vi "PID Get Error (DBL).vi"(0 "setpoint":dbl format="%.2f", 1 "process variable":dbl format="%.2f", 2 "beta":dbl=1.0 format="%.2f", 3 "linearity":dbl=1.0 format="%.2f", 4 "setpoint range":cluster{"setpoint high":dbl, "setpoint low":dbl}={"setpoint high"=100.0, "setpoint low"=0.0} {"setpoint high" format="%.2f"; "setpoint low" format="%.2f"}) -> (5 "error (with beta)":dbl format="%.2f", 6 "error":dbl format="%.2f")   [LabVIEW 2017, in "NI_PID_pid.lvlib"]
doc: "This function calculates the error between the process variable and setpoint value. The error (with beta) output is used for the proportional action and the error output is used for the integral action."
uses:
  <vilib>/addons/control/pid/NI_PID_pid.lvlib
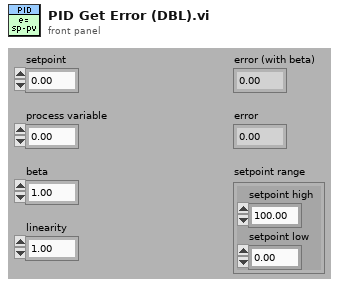
[diagram p1: front panel]
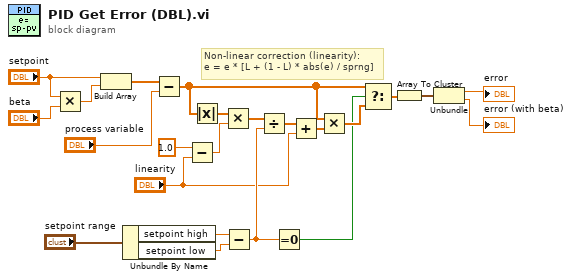
[diagram p0: block diagram]
diagram:
  # "Non-linear correction (linearity):\ne = e * [L + (1 - L) * abs(e) / sprng]"
  n1 = Multiply(x="setpoint", y="beta") -> (x*y=w22:dbl)
  n2 = Build Array("setpoint", w22) -> (w21:dbl[])
  n3 = Unbundle By Name("setpoint range") -> ("setpoint high"=w4:dbl, "setpoint low"=w3:dbl)
  n4 = Subtract(x=w21, y="process variable") -> (x-y=w12:dbl[])
  n5 = Subtract(x=1.0, y="linearity") -> (x-y=w19:dbl)
  n6 = Absolute Value(x=w12) -> (abs(x)=w20:dbl[])
  n7 = Multiply(x=w20, y=w19) -> (x*y=w18:dbl[])
  n8 = Subtract(x=w4, y=w3) -> (x-y=w14:dbl)
  n9 = Divide(x=w18, y=w14) -> (x/y=w17:dbl[])
  n10 = Equal To 0?(x=w14) -> (x = 0?=w10:bool)
  n11 = Add(x=w17, y="linearity") -> (x+y=w16:dbl[])
  n12 = Multiply(x=w12, y=w16) -> (x*y=w11:dbl[])
  n13 = Select(t=w12, s=w10, f=w11) -> (s? t:f=w13:dbl[])
  n14 = Array To Cluster(array=w13) -> (cluster=w15:cluster{"[0]":dbl, "[1]":dbl})
  n15 = Unbundle(w15) -> ("[0]"=→"error":dbl, "[1]"=→"error (with beta)":dbl)
